vi "Compiled Get Node Frames.vi"(6 "Type":T5, 8 "error in (no error)":errorcluster, 9 "Refs in":T4 {"Trigger Refs" format="%.0x"; "Disable Refs" format="%.0x"; "VS Refs" format="%.0x"}, 10 "Cluster":refnum<k21>, 11 "Section Ref in":T2 format="%.0x") -> (0 "error out":errorcluster, 1 "Counter and Protection Frames Properties":T1[](array[typedef]) {"Transmit Trigger Ref" format="%.0x"; "Disable Transmission Ref" format="%.0x"}, 2 "Counter and Protection Frames":T2[](array[typedef]) format="%.0x", 3 "Standard Frames":T6[](array[typedef]), 4 "Refs out":T4 {"Trigger Refs" format="%.0x"; "Disable Refs" format="%.0x"; "VS Refs" format="%.0x"})   [LabVIEW 2023, in "J1939 Addon System Explorer.lvlib"]
uses:
  J1939 Addon System Explorer.lvlib
  <vilib>/NI VeriStand/Custom Device API/Custom Device Item Ref.ctl
  Addon Shared/Types/Outgoing Frame Settings.ctl
  Addon Shared/Types/Outgoing Event Trigger Types.ctl
  SubModules/Frame-Protection-Support/Source/Shared/Types/Exported Frame Type.ctl
  Types/Compiled Refs.ctl
  Addon Shared/Types/Frame.Settings.ctl
  Support Libraries/J1939 Utilities/SubVIs/Convert CAN Arb ID to J1939 ID.vi
  Addon Shared/SubVIs/Constants.vi
  <vilib>/NI VeriStand/Custom Device API/Custom Device API.lvlib
  Addon Shared/J1939 Addon Shared.lvlib
  Support Libraries/J1939 Utilities/J1939 Utilities.lvlib
  SubModules/Frame-Protection-Support/Source/Shared/Protection and Counter Support Shared.lvlib
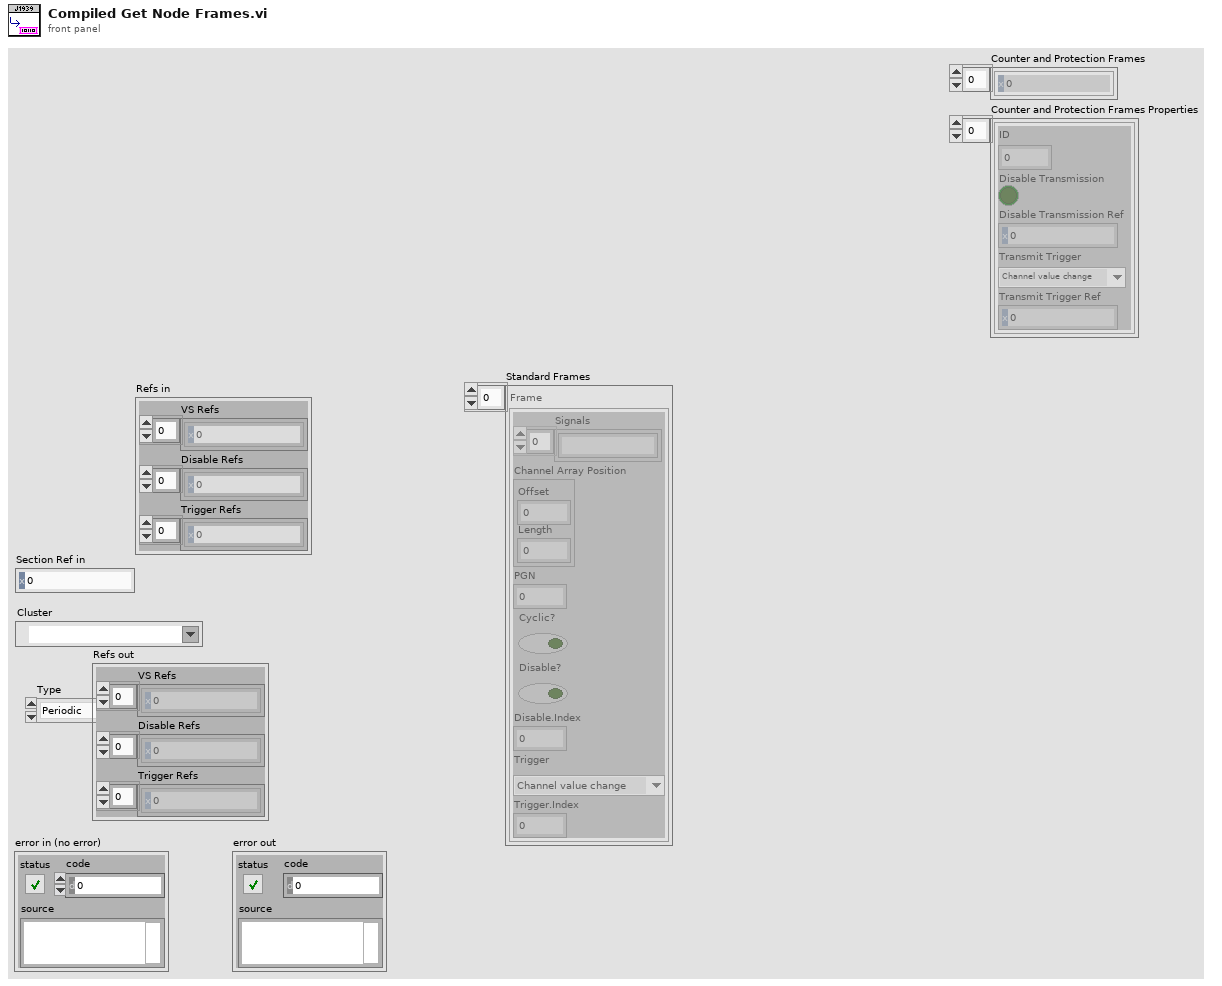
[diagram p1: front panel]
types:
  T1 = typedef "J1939 Addon Shared.lvlib/Frame.Settings.ctl" = cluster{"ID":u32, "Disable Transmission":bool, "Disable Transmission Ref":T2, "Transmit Trigger":T3, "Transmit Trigger Ref":T2}
  T2 = typedef "Custom Device API.lvlib/Custom Device Item Ref.ctl" = u64
  T3 = typedef "J1939 Addon Shared.lvlib/Outgoing Event Trigger Types.ctl" = enum16{"Channel value change", "Trigger channel (not zero)", "Channel value change or trigger channel (not zero)", "Trigger channel (any value change)", "Channel value change or trigger channel (any value change)"}
  T4 = typedef "J1939 Addon System Explorer.lvlib/Compiled Refs.ctl" = cluster{"VS Refs":T2[], "Disable Refs":T2[], "Trigger Refs":T2[]}
  T5 = typedef "Protection and Counter Support Shared.lvlib/Exported Frame Type.ctl" = enum16{"Periodic", "Event", "Periodic/Event"}
  T6 = typedef "J1939 Addon Shared.lvlib/Outgoing Frame Settings.ctl" = cluster{"Signals":string[], "Channel Array Position":cluster{"Offset":u32, "Length":u32}, "PGN":u32, "Cyclic?":bool, "Disable?":bool, "Disable.Index":i32, "Trigger":T3, "Trigger.Index":i32}
  T7 = typedef "Custom Device API.lvlib/Custom Device Item Info.ctl" = cluster{"Name":string, "Is Channel":bool, "GUID":string, "Is Waveform":bool}
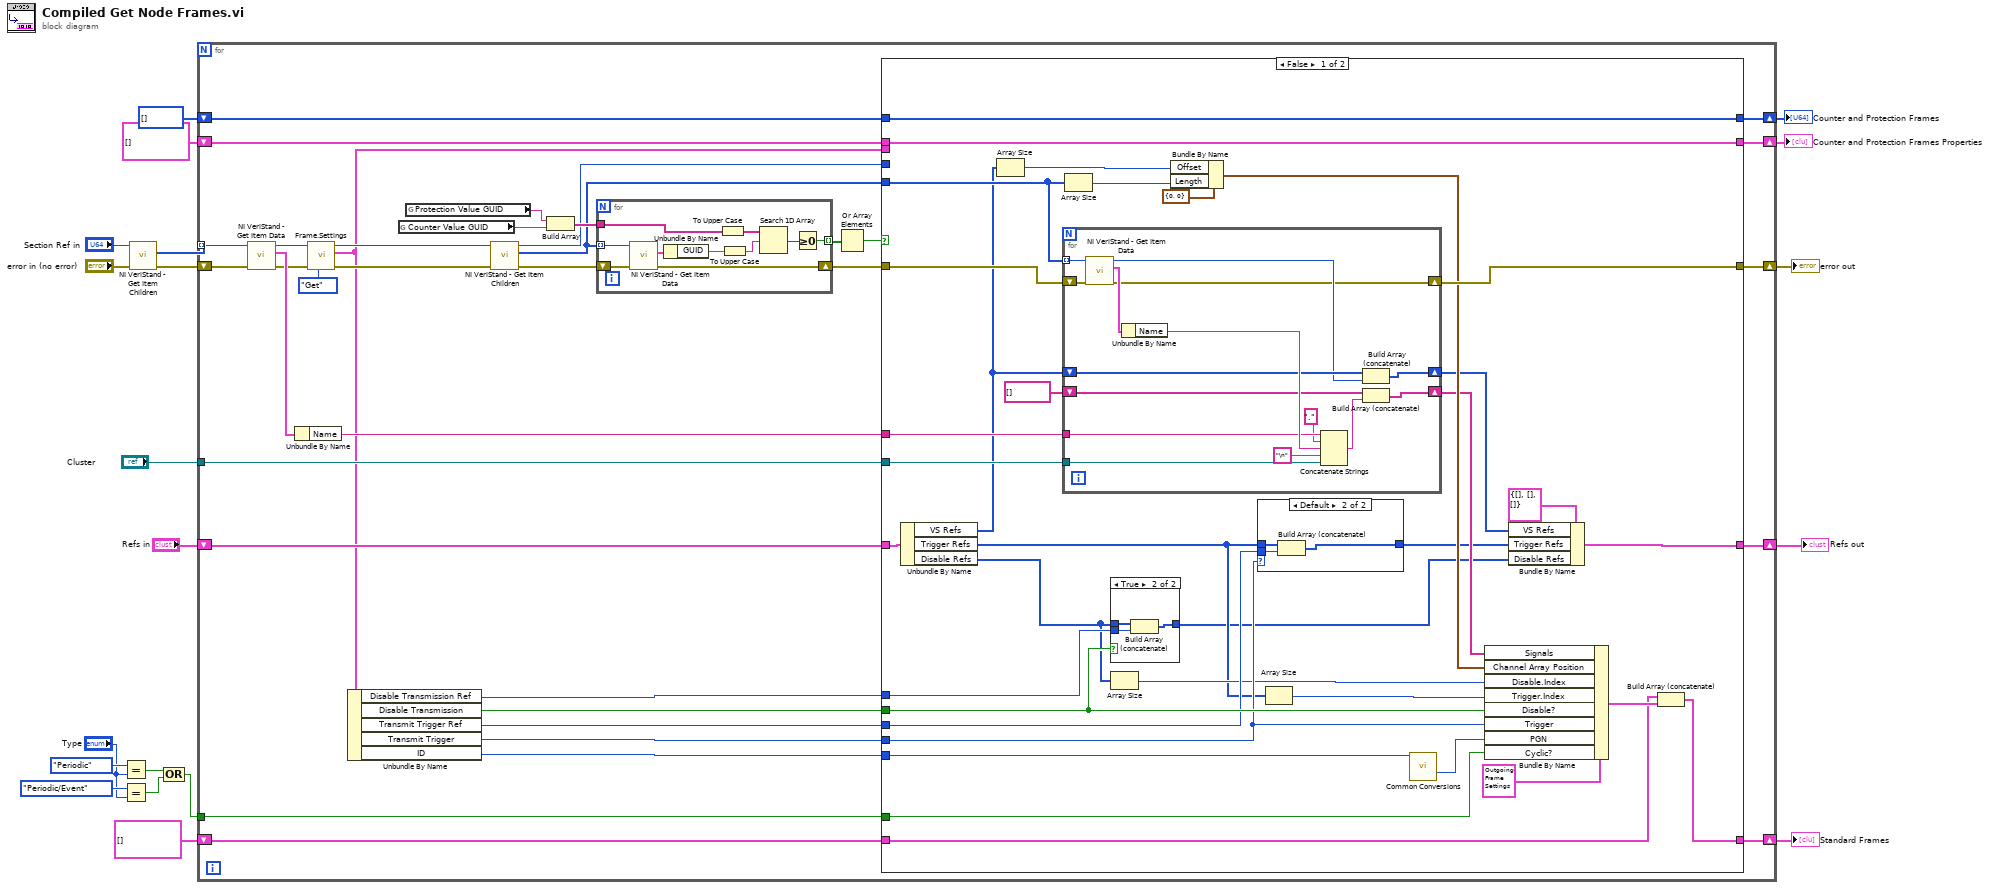
[diagram p0: block diagram]
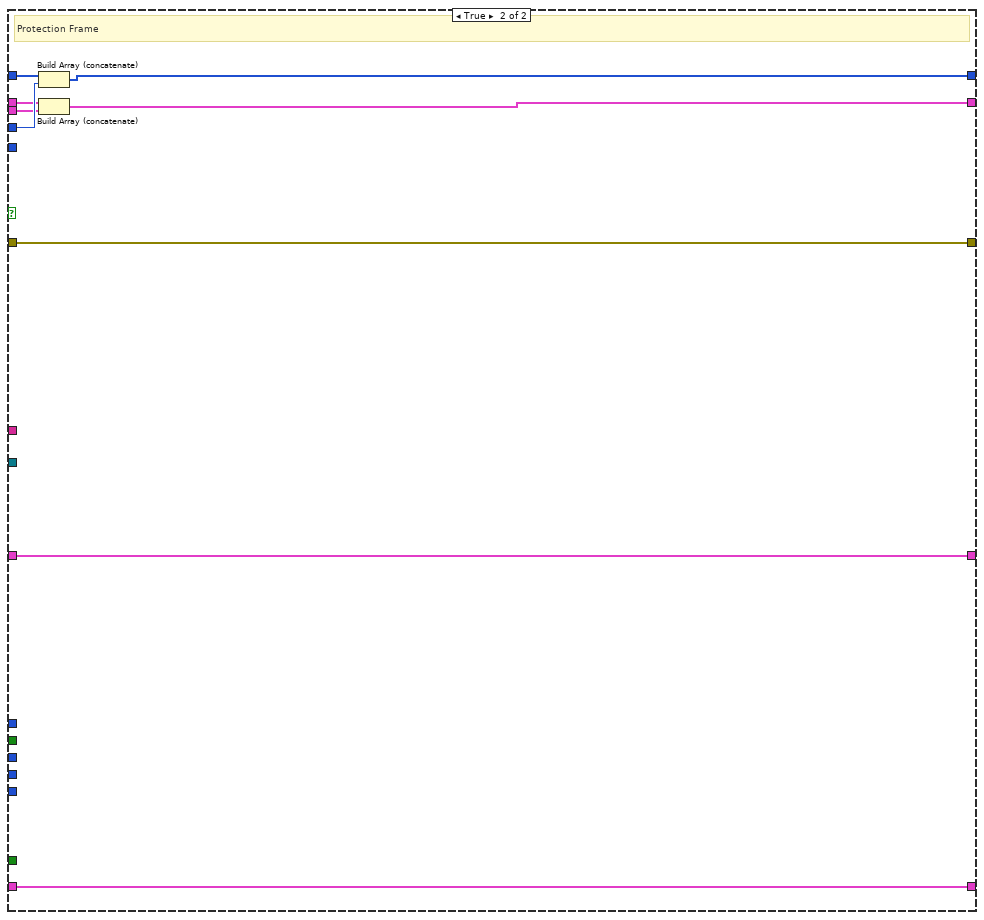
[diagram p4: hidden frame]
diagram:
  n1 = Equal?(x=Exported_Frame_Type."Periodic", y="Type") -> (x = y?=w8:bool)
  n2 = Equal?(x=Exported_Frame_Type."Periodic/Event", y="Type") -> (x = y?=w7:bool)
  n3 = call <vilib>:"NI VeriStand - Get Item Children.vi"("error in (no error)"="error in (no error)", "Item Ref in"="Section Ref in") -> ("error out"=w17:errorcluster, "Child Refs"=w19:T2[])  [unwired: 6 in, 2 out]
  n4 = Compound Arithmetic op=OR(w8, w7) -> (w5:bool)
  n5 = for {
    shift-right: [w47] -> w20
    shift-left: w17 -> [w52]
    tunnel: w19 -> [w53] mode=indexing
    tunnel: "Cluster" -> [w46]
    tunnel: w5 -> [w45]
    shift-right: [w28] -> w13
    shift-left: "Refs in" -> [w29]
    shift-right: [w26] -> w11
    shift-left: T6[] [] -> [w27]
    shift-right: [w25] -> w3
    shift-left: T2[] [] -> [w24]
    shift-right: [w22] -> w1
    shift-left: T1[] [] -> [w21]
    n6 = call <vilib>:"NI VeriStand - Get Item Data.vi"("error in (no error)"=w52, "Item Ref in"=w53) -> ("error out"=w49:errorcluster, "Item Info"=w51:T7, "Item Ref out"=w50:T2)  [unwired: 6 in, 1 out]
    n7 = Unbundle By Name(w51) -> ("Name"=w48:string)
    n8 = call "Frame.Settings.vi"("Action"=enum8{"Get", "Set"}."Get", "error in (no error)"=w49, "Item Ref in"=w50) -> ("error out"=w55:errorcluster, "Frame.Settings"=w23:T1, "Item Ref out"=w54:T2)  [unwired: 6 in]
    n9 = Unbundle By Name(w23) -> ("Disable Transmission Ref"=w41:T2, "Disable Transmission"=w42:bool, "Transmit Trigger Ref"=w40:T2, "Transmit Trigger"=w39:T3, "ID"=w43:u32)
    n10 = global read "Constants.vi" "Counter Value GUID"() -> (w38:string)
    n11 = global read "Constants.vi" "Protection Value GUID"() -> (w37:string)
    n12 = call <vilib>:"NI VeriStand - Get Item Children.vi"("error in (no error)"=w55, "Item Ref in"=w54) -> ("error out"=w34:errorcluster, "Child Refs"=w32:T2[], "Item Ref out"=w30:T2)  [unwired: 6 in, 1 out]
    n13 = Build Array(w37, w38) -> (w36:string[])
    n14 = for {
      tunnel: w32 -> [w130] mode=indexing
      tunnel: w36 -> [w128]
      tunnel: [w124] -> w35 mode=indexing
      shift-right: [w123] -> w33
      shift-left: w34 -> [w131]
      n15 = call <vilib>:"NI VeriStand - Get Item Data.vi"("error in (no error)"=w131, "Item Ref in"=w130) -> ("error out"=w123:errorcluster, "Item Info"=w132:T7)  [unwired: 6 in, 2 out]
      n16 = Unbundle By Name(w132) -> ("GUID"=w129:string)
      n17 = To Upper Case(1:w128) -> (0:w127:string[])
      n18 = To Upper Case(1:w129) -> (0:w126:string)
      n19 = Search 1D Array(1D array=w127, element=w126) -> (index of element=w125:i32)  [unwired: 1 in]
      n20 = Greater Or Equal To 0?(x=w125) -> (x >= 0?=w124:bool)
    }
    n21 = Or Array Elements(Boolean array=w35) -> (logical OR=w31:bool)
    n22 = case shown="False" w31 {
      tunnel: w48 -> [w88 _]
      tunnel: [w87 w122] -> w47
      tunnel: w46 -> [w86 _]
      tunnel: w45 -> [w82 _]
      tunnel: w43 -> [w79 _]
      tunnel: w42 -> [w78 _]
      tunnel: w41 -> [w77 _]
      tunnel: w40 -> [w76 _]
      tunnel: w39 -> [w75 _]
      tunnel: w33 -> [w72 w122]
      tunnel: w32 -> [w71 _]
      tunnel: w30 -> [_ w118]
      tunnel: w29 -> [w69 w121]
      tunnel: [w61 w121] -> w28
      tunnel: w27 -> [w59 w120]
      tunnel: [w58 w120] -> w26
      tunnel: [w57 w117] -> w25
      tunnel: w24 -> [w57 w119]
      tunnel: w23 -> [_ w116]
      tunnel: [w56 w115] -> w22
      tunnel: w21 -> [w56 w114]
      frame False {
        n23 = Unbundle By Name(w69) -> ("VS Refs"=w66:T2[], "Trigger Refs"=w67:T2[], "Disable Refs"=w68:T2[])
        n24 = Array Size(array=w66) -> (size(s)=w70:i32)
        n25 = for {
          shift-right: [w102] -> w87
          shift-left: w72 -> [w112]
          tunnel: w71 -> [w113] mode=indexing
          shift-right: [w107] -> w64
          shift-left: w66 -> [w108]
          tunnel: w88 -> [w106]
          tunnel: w86 -> [w104]
          shift-right: [w109] -> w80
          shift-left: string[] [] ("Signals") -> [w103]
          n26 = call <vilib>:"NI VeriStand - Get Item Data.vi"("error in (no error)"=w112, "Item Ref in"=w113) -> ("error out"=w102:errorcluster, "Item Info"=w111:T7, "Item Ref out"=w105:T2)  [unwired: 6 in, 1 out]
          n27 = Unbundle By Name(w111) -> ("Name"=w110:string)
          n28 = Concatenate Strings(w106, "." ("string"), w110, "\n" ("string"), w104) -> (w99:string)
          n29 = Build Array (concatenate)(w108, w105) -> (w107:T2[])
          n30 = Build Array (concatenate)(w103, w99) -> (w109:string[])
        }
        n31 = Array Size(array=w71) -> (size(s)=w89:i32)
        n32 = case shown="True" w78 {
          tunnel: w68 -> [w95 w98]
          tunnel: w77 -> [_ w97]
          tunnel: [w95 w96] -> w62
          frame False {
          }
          frame True {
            n33 = Build Array (concatenate)(w98, w97) -> (w96:T2[])
          }
        }
        n34 = Array Size(array=w68) -> (size(s)=w73:i32)
        n35 = Bundle By Name(cluster=cluster{"Offset":u32, "Length":u32} {"Offset"=0, "Length"=0} ("Channel Array Position"), "Offset"=w70, "Length"=w89) -> (w85:cluster{"Offset":u32, "Length":u32})
        n36 = case shown="Default" w75 {
          tunnel: w67 -> [w91 w94]
          tunnel: w76 -> [_ w93]
          tunnel: [w91 w92] -> w63
          frame "Channel value change" {
          }
          frame Default {
            n37 = Build Array (concatenate)(w94, w93) -> (w92:T2[])
          }
        }
        n38 = Array Size(array=w67) -> (size(s)=w74:i32)
        n39 = call-poly "Common Conversions.vi"("Arb ID"=w79) -> ("PGN"=w83:u32)  [unwired: 11 in, 3 out]
        n40 = Bundle By Name(cluster=T6 {"Signals"=[], "Channel Array Position"={"Offset"=0, "Length"=0}, "PGN"=0, "Cyclic?"=FALSE, "Disable?"=FALSE, "Disable.Index"=0, "Trigger"=enum."Channel value change", "Trigger.Index"=0} ("Frame"), "Signals"=w80, "Channel Array Position"=w85, "Disable.Index"=w73, "Trigger.Index"=w74, "Disable?"=w78, "Trigger"=w75, "PGN"=w83, "Cyclic?"=w82) -> (w60:T6)
        n41 = Bundle By Name(cluster=T4 {"VS Refs"=[], "Disable Refs"=[], "Trigger Refs"=[]} ("Refs in"), "VS Refs"=w64, "Trigger Refs"=w63, "Disable Refs"=w62) -> (w61:T4)
        n42 = Build Array (concatenate)(w59, w60) -> (w58:T6[])
      }
      frame True {
        # "Protection Frame"
        n43 = Build Array (concatenate)(w119, w118) -> (w117:T2[])
        n44 = Build Array (concatenate)(w114, w116) -> (w115:T1[])
      }
    }
  }
  "error out" <- w20
  "Standard Frames" <- w11
  "Refs out" <- w13
  "Counter and Protection Frames" <- w3
  "Counter and Protection Frames Properties" <- w1
